vi "Configure Safety Trigger.vi"() -> ()   [LabVIEW 2025, in "Rigol.lvlib"]
uses:
  Rigol.lvlib
panel:
  out "VISA resource name out":refnum<visa-resource-name>
  out "value out":errorcluster
  in  "error in (no error)":errorcluster
  in  "VISA resource name":refnum<visa-resource-name>
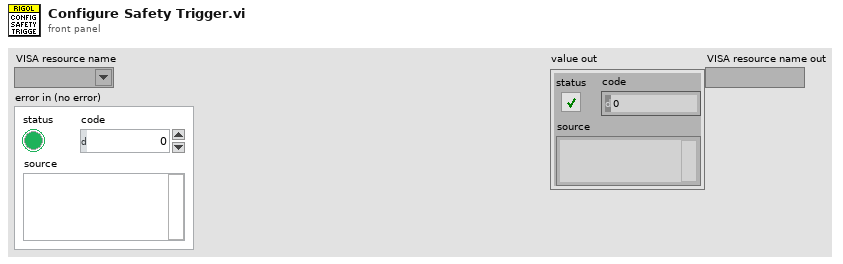
[diagram p1: front panel]
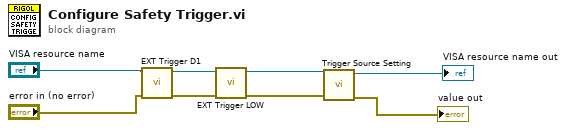
[diagram p0: block diagram]
diagram:
  n1 = call "EXT Trigger D1.vi"("error in (no error)"="error in (no error)", "VISA resource name"="VISA resource name") -> ("value out"=w7:errorcluster, "VISA resource name out"=w4:refnum<visa-resource-name>)  [unwired: 8 in]
  n2 = call "EXT Trigger LOW.vi"("error in (no error)"=w7, "VISA resource name"=w4) -> ("value out"=w8:errorcluster, "VISA resource name out"=w3:refnum<visa-resource-name>)  [unwired: 8 in]
  n3 = call "Trigger Source Setting.vi"("error in (no error)"=w8, "VISA resource name"=w3) -> ("value out"=→"value out":errorcluster, "VISA resource name out"=→"VISA resource name out":refnum<visa-resource-name>)  [unwired: 8 in]
